vi "SENS_SEGM_SWE_TIME.vi"(0 "VISA IN":refnum<visa-resource-name>, 1 "Segment":i32, 2 "Sweep Time(sec)":i32, 5 "error in":errorcluster, 7 "Channel":i32) -> (14 "VISA Out":refnum<visa-resource-name>, 19 "error out":errorcluster)   [LabVIEW 2018, in "PNA-X.lvlib"]
doc: "SENSe<cnum>:SEGMent<snum>:SWEep:TIME <num> \n(Read-Write) Sets the time the analyzer takes to sweep the specified sweep segment. \nParameters \n<cnum> Any existing channel number. If unspecified, value is set to 1 \n<snum> Any existing segment number. \n<num> Sweep time in seconds. Choose a number between 0 and 100 \nNote: This command will accept MIN or MAX instead of a numeric \nparameter. See SCPI Syntax for more information. \nExamples SENS:SEGM:SWE:TIME 1ms \nsense2:segment2:sweep:time .001 \nQuery Syntax SENSe<cnum>:SEGMent<snum>:SWEep:TIME? \nReturn Type Numeric \nDefault Not Applicable"
uses:
  PNA-X.lvlib
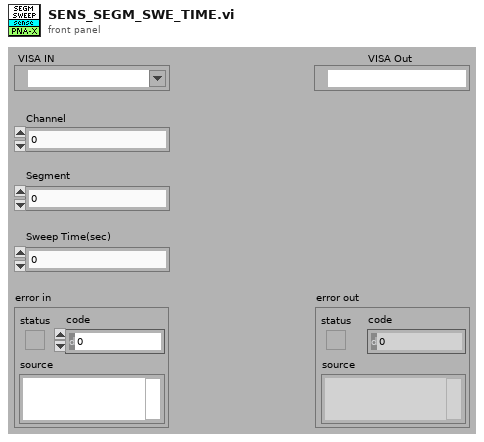
[diagram p1: front panel]
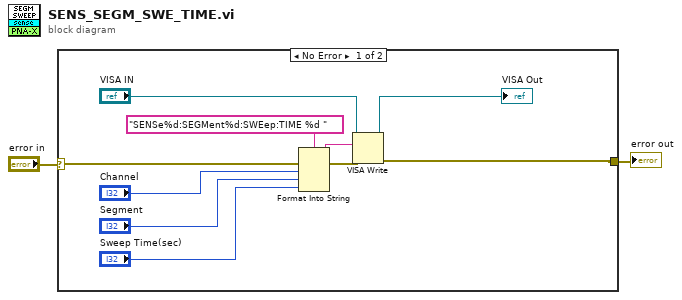
[diagram p0: block diagram]
diagram:
  n1 = case shown="No Error" "error in" {
    selector: "error in" -> [w12 w13]
    tunnel: [w7 w13] -> w1
    frame No Error {
      n2 = Format Into String(format string="SENSe%d:SEGMent%d:SWEep:TIME %d " ("Cmdline"), error in=w12, "Channel", "Segment", "Sweep Time(sec)") -> (resulting string=w10:string, error out=w11:errorcluster)  [unwired: 1 in]
      n3 = VISA Write(VISA resource name="VISA IN", write buffer=w10, error in (no error)=w11) -> (VISA resource name out=→"VISA Out":refnum<visa-resource-name>, error out=w7:errorcluster)  [unwired: 1 out]
    }
    frame Error {
    }
  }
  "error out" <- w1
